vi "enumerate devices.vi"(8 "error in (no error)":errorcluster, 10 "hints":string, 11 "enumerate_flags":i32) -> (0 "error out":errorcluster, 3 "function return":u32)   [LabVIEW 2012, in "libximc.lvlib"]
doc: "device_enumeration_t XIMC_API enumerate_devices(int enumerate_flags, const char *hints);"
uses:
  libximc.lvlib
  libximc.dll
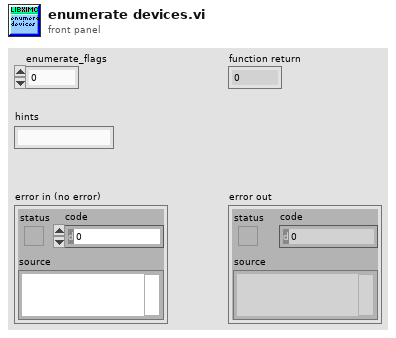
[diagram p1: front panel]
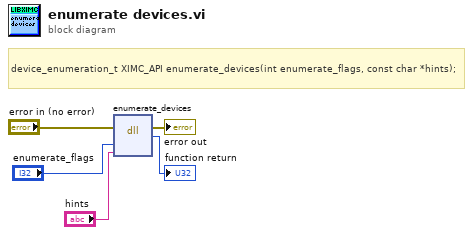
[diagram p0: block diagram]
diagram:
  # "device_enumeration_t XIMC_API enumerate_devices(int enumerate_flags, const char *hints);"
  n1 = dll-call lib="C:/Users/user/Desktop/labview-2.9.11-gen/libximc.*" fn="enumerate_devices"(error in="error in (no error)", "enumerate_flags"="enumerate_flags", "hints"="hints") -> (error out=→"error out":errorcluster, →"function return":u32)  [unwired: 4 in, 1 out]
